vi "SET_HEADING_ONEWHEEL.vi"(10 "argv":string[](array[string]), 11 "args":u8) -> ()   [LabVIEW 2015]
uses:
  Team Code/Robot Global Data.vi
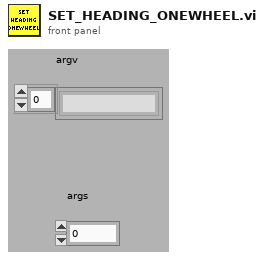
[diagram p1: front panel]
types:
  T1 = typedef "WPI_GyroDevRef.ctl" = cluster{"DevStatus":errorcluster, "Analog Channel":T2, "Offset":dbl, "Gain (VoltsPerDegree/Second)":dbl}
  T2 = typedef "FPGA_AIChannel.ctl" = enum8{"AI 0", "AI 1", "AI 2", "AI 3", "AI MXP 0", "AI MXP 1", "AI MXP 2", "AI MXP 3", "Invalid"}
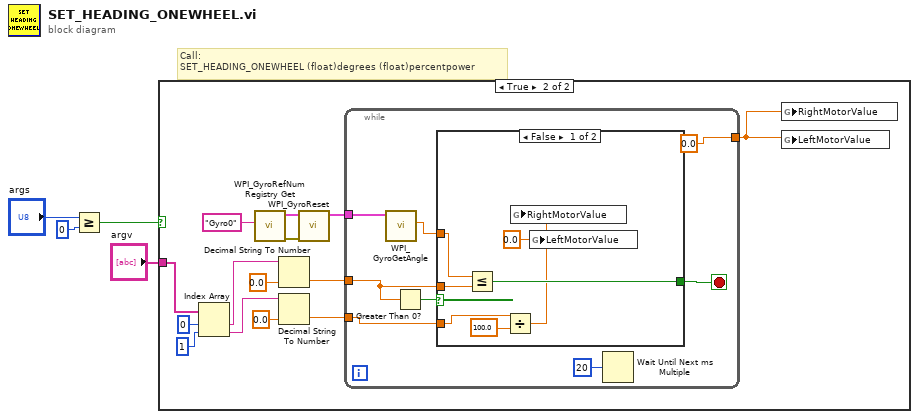
[diagram p0: block diagram]
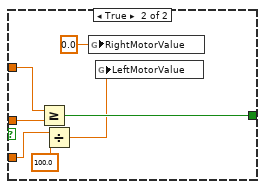
[diagram p3: hidden frame]
diagram:
  # "Call:\nSET_HEADING_ONEWHEEL (float)degrees (float)percentpower"
  n1 = Greater Or Equal?(x="args", y=u8 0) -> (x >= y?=w4:bool)
  n2 = case shown="True" w4 {
    tunnel: "argv" -> [_ w13]
    frame False {
    }
    frame True {
      n3 = Index Array(array=w13, index #1=0 ("index"), index #2=1 ("index")) -> (element #1=w9:string, element #2=w6:string)
      n4 = call <vilib>:"WPI_GyroRefNum Registry Get.vi"("refnum name"="Gyro0") -> ("error out"=w16:errorcluster, "GyroDevRef"=w14:T1)  [unwired: 9 in]
      n5 = Decimal String To Number(string=w9, default (0L)=0.0 ("default (0 I32)")) -> (number=w8:dbl)  [unwired: 2 out]
      n6 = Decimal String To Number(string=w6, default (0L)=0.0 ("default (0 I32)")) -> (number=w5:dbl)  [unwired: 2 out]
      n7 = call <vilib>:"WPI_GyroReset.vi"("error in (no error)"=w16, "GyroDevRef"=w14) -> ("GyroDevRef"=w15:T1)  [unwired: 8 in, 1 out]
      n8 = while {
        tunnel: w8 -> [w21]
        tunnel: w15 -> [w24]
        tunnel: [0.0 ("LeftMotorValue")] -> w17
        tunnel: w5 -> [w20]
        stop <- w23 stop-if-true
        n9 = call <vilib>:"WPI_GyroGetAngle.vi"("GyroDevRef"=w24) -> ("Angle"=w19:dbl)  [unwired: 7 in, 3 out]
        n10 = Greater Than 0?(x=w21) -> (x > 0?=w25:bool)
        n11 = case shown="False" w25 {
          tunnel: [w33 w40] -> w23
          tunnel: w21 -> [w32 w39]
          tunnel: w20 -> [w30 w35]
          tunnel: w19 -> [w28 w36]
          frame False {
            n12 = Less Or Equal?(x=w28, y=w32) -> (x <= y?=w33:bool)
            n13 = Divide(x=w30, y=100.0) -> (x/y=w31:dbl)
            n14 = global write "Robot Global Data.vi" "RightMotorValue"(w31) -> ()
            n15 = global write "Robot Global Data.vi" "LeftMotorValue"(0.0 ("LeftMotorValue")) -> ()
          }
          frame True {
            n16 = Greater Or Equal?(x=w36, y=w39) -> (x >= y?=w40:bool)
            n17 = Divide(x=w35, y=100.0) -> (x/y=w38:dbl)
            n18 = global write "Robot Global Data.vi" "RightMotorValue"(0.0 ("LeftMotorValue")) -> ()
            n19 = global write "Robot Global Data.vi" "LeftMotorValue"(w38) -> ()
          }
        }
        n20 = Wait Until Next ms Multiple(millisecond multiple=u32 20) -> ()  [unwired: 1 out]
      }
      n21 = global write "Robot Global Data.vi" "RightMotorValue"(w17) -> ()
      n22 = global write "Robot Global Data.vi" "LeftMotorValue"(w17) -> ()
    }
  }
